vi "Get Paragraphs.vi"(8 "error in (no error)":errorcluster, 11 "xwpfHeader in":refnum<class "xwpfHeader_Footer.lvclass">) -> (0 "error out":errorcluster, 2 "Paragraphs":refnum<class "xwpfParagraph.lvclass">[](array[class]), 3 "xwpfHeader out":refnum<class "xwpfHeader_Footer.lvclass">)   [LabVIEW 2017, in "Word_Specific.lvlib" / "xwpfHeader_Footer.lvclass"]
uses:
  xwpfHeader_Footer.lvclass
  xwpfParagraph/xwpfParagraph.lvclass
  xwpfHeader_Footer.lvclass/xwpfHeader_Footer.ctl
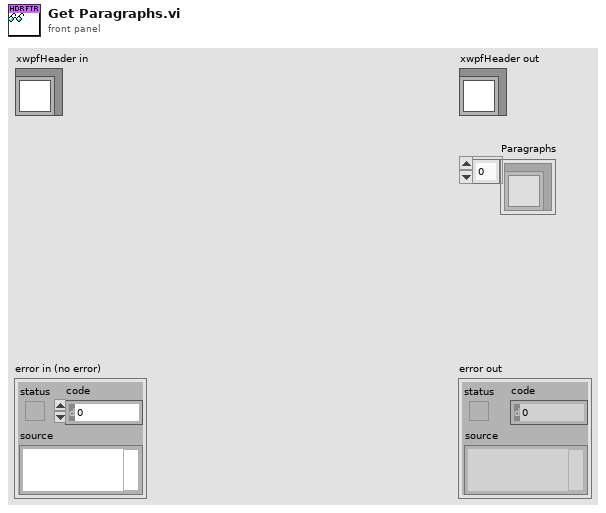
[diagram p1: front panel]
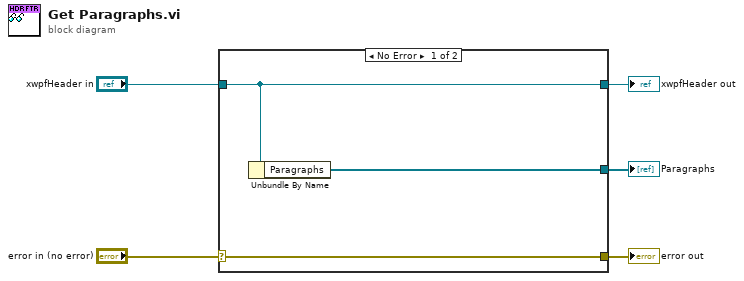
[diagram p0: block diagram]
diagram:
  n1 = case shown="No Error" "error in (no error)" {
    selector: "error in (no error)" -> [w8 w9]
    tunnel: [w8 w9] -> w4
    tunnel: [w7 w10] -> w2
    tunnel: "xwpfHeader in" -> [w7 w10]
    tunnel: [w6 _] -> w1
    frame No Error {
      n2 = Unbundle By Name(w7) -> ("Paragraphs"=w6:refnum<class "xwpfParagraph.lvclass">[])
    }
    frame Error {
    }
  }
  "error out" <- w4
  "xwpfHeader out" <- w2
  "Paragraphs" <- w1
